vi "Triangulate Spark.vi"(3 "timings":dbl[](array[numeric]), 4 "cavity length (s)":dbl, 5 "cavity diameter (s)":dbl) -> (0 "coordinates_prime":T1, 1 "coordinates":cluster{"x":dbl, "y":dbl, "z":dbl})   [LabVIEW 2012]
panel:
  out "z^2":dbl
  out "y^2":dbl
  out "x^2":dbl
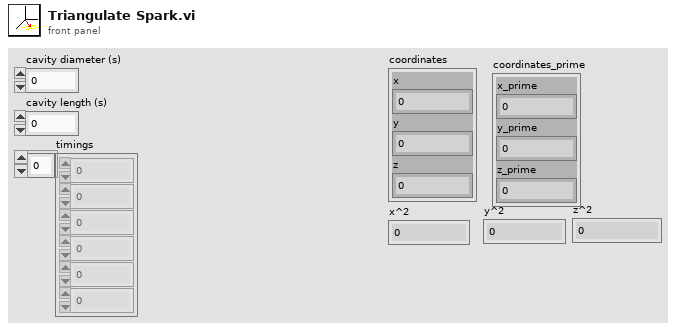
[diagram p1: front panel]
types:
  T1 = cluster{"x_prime":dbl, "y_prime":dbl, "z_prime":dbl}
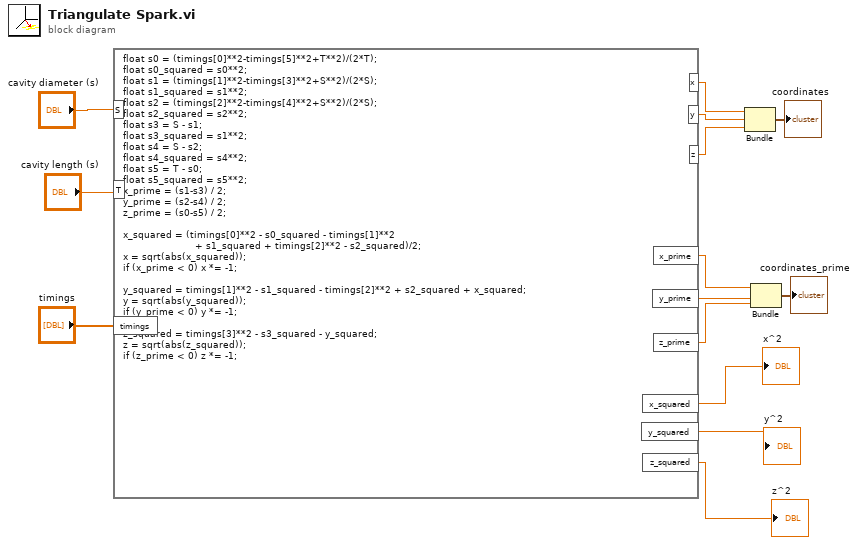
[diagram p0: block diagram]
diagram:
  n1 = formula code="float s0 = (timings[0]**2-timings[5]**2+T**2)/(2*T);\nfloat s0_squared = s0**2;\nfloat s1 = (timings[1]**2-timings[3]**2+S**2)/(2*S);\nfloat s1_squared = s1**2;\nfloat s2 = (timings[2]**2-timings[4]**2+S**2)/(2*S);\nfloat s2_squared = s2**2;\nfloat s3 = S - s1;\nfloat s3_squared = s1**2;\nfloat s4 = S - s2;\nfloat s4_squared = s4**2;\nfloat s5 = T - s0;\nfloat s5_squared = s5**2;\nx_prime = (s1-s3) / 2;\ny_prime = (s2-s4) / 2;\nz_prime = (s0-s5) / 2;\n\nx_squared = (timings[0]**2 - s0_squared - timings[1]**2\n                        + s1_squared + timings[2]**2 - s2_squared)/2;\nx = sqrt(abs(x_squared));\nif (x_prime < 0) x *= -1;\n \ny_squared = timings[1]**2 - s1_squared - timings[2]**2 + s2_squared + x_squared;\ny = sqrt(abs(y_squared));\nif (y_prime < 0) y *= -1;\n\nz_squared = timings[3]**2 - s3_squared - y_squared;\nz = sqrt(abs(z_squared));\nif (z_prime < 0) z *= -1;"("S"="cavity diameter (s)", "timings"="timings", "T"="cavity length (s)") -> ("x"=w11:dbl, "y"=w10:dbl, "z"=w9:dbl, "x_prime"=w8:dbl, "y_prime"=w7:dbl, "z_prime"=w6:dbl, "x_squared"=→"x^2":dbl, "y_squared"=→"y^2":dbl, "z_squared"=→"z^2":dbl)
  n2 = Bundle("x"=w11, "y"=w10, "z"=w9) -> (→"coordinates":cluster{"x":dbl, "y":dbl, "z":dbl})  [unwired: 1 in]
  n3 = Bundle("x_prime"=w8, "y_prime"=w7, "z_prime"=w6) -> (→"coordinates_prime":T1)  [unwired: 1 in]
